vi "timer.vi"(8 "error in":errorcluster, 10 "limit":dbl, 11 "timerstat":T1) -> (0 "error out":errorcluster, 2 "in limit":bool, 3 "elapsed":dbl)   [LabVIEW 2015]
uses:
  controls/timerstatus.ctl
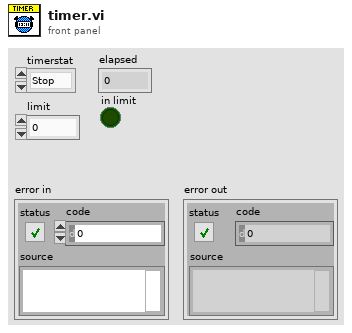
[diagram p1: front panel]
types:
  T1 = typedef "timerstatus.ctl" = enum16{"Stop", "Start"}
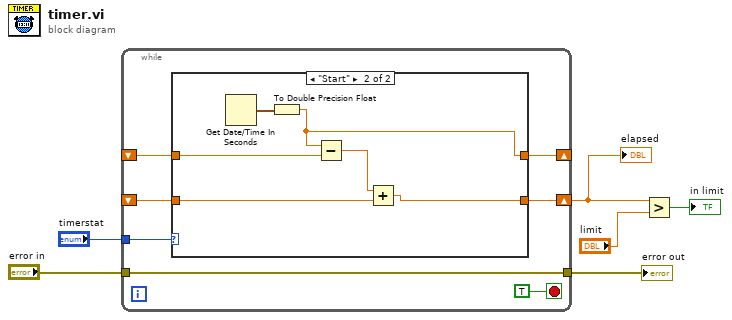
[diagram p0: block diagram]
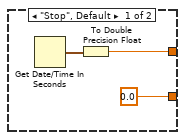
[diagram p2: hidden frame]
diagram:
  n1 = while {
    tunnel: "timerstat" -> [w12]
    shift-right: [w10] -> w4
    shift-left: _ -> [w8]
    shift-right: [w11] -> _
    shift-left: _ -> [w9]
    tunnel: "error in" -> [w7]
    tunnel: [w7] -> w1
    stop <- TRUE stop-if-true
    n2 = case shown="\"Start\"" w12 {
      tunnel: [w15 w17] -> w11
      tunnel: [0.0 w18] -> w10
      tunnel: w9 -> [_ w21]
      tunnel: w8 -> [_ w19]
      frame "Stop", Default {
        n3 = Get Date/Time In Seconds() -> (seconds since 1Jan1904=w16:timestamp)
        n4 = To Double Precision Float(number=w16) -> (double precision float=w15:dbl)
      }
      frame "Start" {
        n5 = Get Date/Time In Seconds() -> (seconds since 1Jan1904=w22:timestamp)
        n6 = To Double Precision Float(number=w22) -> (double precision float=w17:dbl)
        n7 = Subtract(x=w17, y=w21) -> (x-y=w20:dbl)
        n8 = Add(x=w20, y=w19) -> (x+y=w18:dbl)
      }
    }
  }
  "elapsed" <- w4
  "error out" <- w1
  n9 = Greater?(x=w4, y="limit") -> (0:→"in limit":bool)
